vi "create folder path.vi"(8 "error in (no error)":errorcluster, 11 "Cascade in":refnum<class "Cascade.lvclass">) -> (0 "error out":errorcluster, 2 "dup path":path, 3 "Cascade out":refnum<class "Cascade.lvclass">)   [LabVIEW 2012, in "Cascade.lvclass"]
uses:
  Cascade.lvclass
  Cascade.lvclass/Cascade.ctl
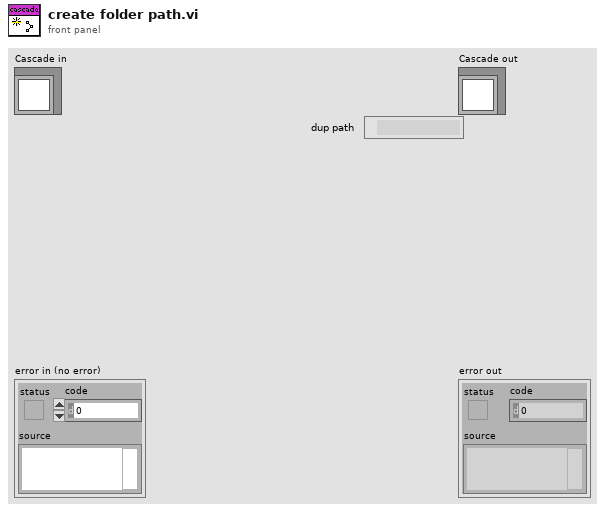
[diagram p1: front panel]
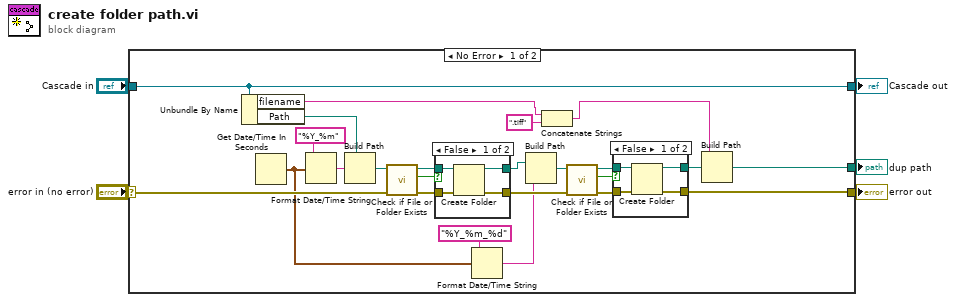
[diagram p0: block diagram]
diagram:
  n1 = case shown="No Error" "error in (no error)" {
    selector: "error in (no error)" -> [w24 w43]
    tunnel: [w11 w43] -> w4
    tunnel: [w29 w42] -> w2
    tunnel: "Cascade in" -> [w29 w42]
    tunnel: [w10 _] -> w1
    frame No Error {
      n2 = Unbundle By Name(w29) -> ("filename"=w7:string, "Path"=w25:path)
      n3 = Get Date/Time In Seconds() -> (seconds since 1Jan1904=w15:timestamp)
      n4 = Format Date/Time String(time format string (%c)="%Y_%m", seconds (now)=w15) -> (date/time string=w27:string)  [unwired: 1 in]
      n5 = Build Path(base path=w25, name or relative path=w27) -> (appended path=w28:path)
      n6 = call <vilib>:"Check if File or Folder Exists.vi"("error in (no error)"=w24, "path"=w28) -> ("error out"=w18:errorcluster, "file or folder exists?"=w16:bool, "dup path"=w17:path)  [unwired: 7 in]
      n7 = case shown="False" w16 {
        tunnel: w18 -> [w39 w41]
        tunnel: w17 -> [w38 w40]
        tunnel: [w37 w41] -> w22
        tunnel: [w36 w40] -> w23
        frame False {
          n8 = Create Folder(path (use dialog)=w38, error in=w39) -> (created path=w36:path, error out=w37:errorcluster)  [unwired: 1 in, 1 out]
        }
        frame True {
        }
      }
      n9 = Format Date/Time String(time format string (%c)="%Y_%m_%d", seconds (now)=w15) -> (date/time string=w20:string)  [unwired: 1 in]
      n10 = Build Path(base path=w23, name or relative path=w20) -> (appended path=w19:path)
      n11 = Concatenate Strings(w7, ".tiff" ("string")) -> (w6:string)
      n12 = call <vilib>:"Check if File or Folder Exists.vi"("error in (no error)"=w22, "path"=w19) -> ("error out"=w13:errorcluster, "file or folder exists?"=w12:bool, "dup path"=w14:path)  [unwired: 7 in]
      n13 = case shown="False" w12 {
        tunnel: w13 -> [w33 w35]
        tunnel: w14 -> [w32 w34]
        tunnel: [w31 w35] -> w11
        tunnel: [w30 w34] -> w9
        frame False {
          n14 = Create Folder(path (use dialog)=w32, error in=w33) -> (created path=w30:path, error out=w31:errorcluster)  [unwired: 1 in, 1 out]
        }
        frame True {
        }
      }
      n15 = Build Path(base path=w9, name or relative path=w6) -> (appended path=w10:path)
    }
    frame Error {
    }
  }
  "error out" <- w4
  "Cascade out" <- w2
  "dup path" <- w1
